vi "File IO Test.vi"() -> ()   [LabVIEW 2019]
panel:
  out "Equal!":bool
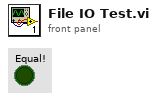
[diagram p1: front panel]
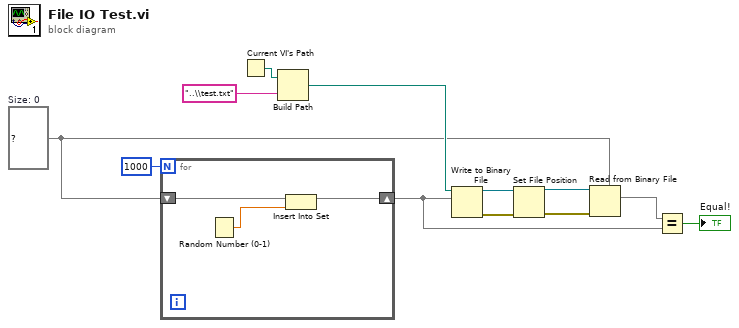
[diagram p0: block diagram]
diagram:
  w4 = set{dbl} {}  # Size: 0
  n1 = for {
    N: 1000 -> [_]
    shift-right: [w13] -> w2
    shift-left: w4 -> [w14]
    n2 = Random Number (0-1)() -> (number: 0 to 1=w15:dbl)
    n3 = Insert Into Set(10:w15, 11:w14) -> (3:w13:set{dbl})  [unwired: 1 out]
  }
  n4 = Current VI's Path() -> (path=w11:path)
  n5 = Build Path(base path=w11, name or relative path="..\\test.txt") -> (appended path=w9:path)
  n6 = Write to Binary File(file (use dialog)=w9, data=w2) -> (refnum out=w8:refnum<file>, error out=w7:errorcluster)  [unwired: 4 in, 1 out]
  n7 = Set File Position(refnum=w8, error in=w7) -> (refnum out=w6:refnum<file>, error out=w5:errorcluster)  [unwired: 2 in]
  n8 = Read from Binary File(5:w4, 8:w5, 11:w6) -> (2:w3:set{dbl})  [unwired: 3 in, 3 out]
  n9 = Equal?(x=w3, y=w2) -> (x = y?=→"Equal!":bool)
